vi "Talker.vi"(0 "Divide in":refnum<class "Divide.lvclass">, 5 "Subpanel Ref":refnum<vi>, 11 "Error In":errorcluster) -> (4 "Divide out":refnum<class "Divide.lvclass">, 15 "Error Out":errorcluster)   [LabVIEW 2020, in "Divide.lvclass"]
doc: "Method to call the UI Method. This will pass the object to the UI Method which will do the operation and return the object to the main vi."
uses:
  Divide.lvclass
  UI.vi
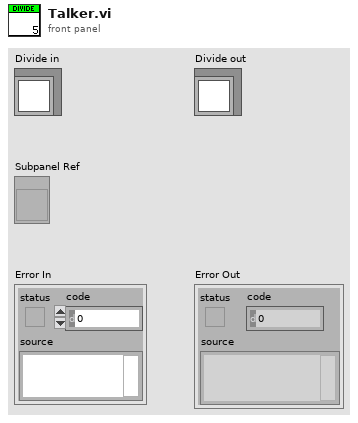
[diagram p1: front panel]
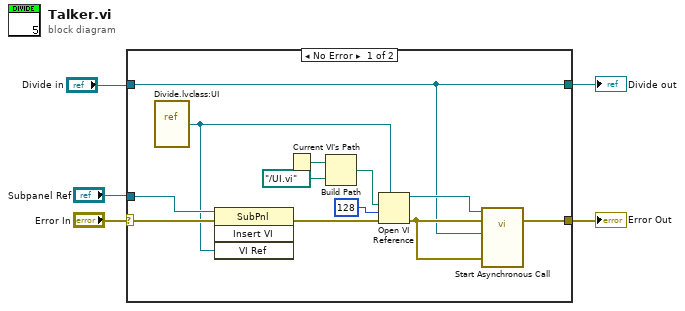
[diagram p0: block diagram]
diagram:
  n1 = case shown="No Error" "Error In" {
    selector: "Error In" -> [w15 w19]
    tunnel: [w10 w19] -> w4
    tunnel: [w11 w18] -> w2
    tunnel: "Divide in" -> [w11 w18]
    tunnel: "Subpanel Ref" -> [w13 _]
    frame No Error {
      n2 = vi-ref "Divide.lvclass:UI.vi"() -> (w9:refnum<vi>)
      n3 = invoke on="Invoke Node" class="SubPnl" method="Insert VI"(reference=w13, error in=w15, "VI Ref"=w9) -> (error out=w14:errorcluster)  [unwired: 1 in, 3 out]
      n4 = Current VI's Path() -> (path=w8:path)
      n5 = Build Path(base path=w8, name or relative path=path "../UI.vi") -> (appended path=w6:path)
      n6 = Open VI Reference(type specifier VI Refnum (for type only)=w9, vi path=w6, options=128, error in (no error)=w14) -> (vi reference=w12:refnum<vi>, error out=w17:errorcluster)  [unwired: 2 in]
      n7 = call-by-ref "Start Asynchronous Call"(reference=w12, error in=w17, "Divide in"=w11, "Error In"=w17) -> (error out=w10:errorcluster)  [unwired: 11 in, 4 out]
    }
    frame Error {
    }
  }
  "Divide out" <- w2
  "Error Out" <- w4
